vi "Reports_GetAllRequestsData.vi"(8 "error in (no error)":errorcluster, 11 "Refnum in":T1) -> (0 "error out":errorcluster, 2 "Array":string[][](array[string]), 3 "Refnum Out":T1)   [LabVIEW 2013, in "FIRST Reports.lvlib"]
uses:
  FIRST Reports.lvlib
  <vilib>/addons/database/Connection.llb/Conn ObjectReference.ctl
  Backend/source/VI Source/FRCts20_Backend_Engine.lvlib
  <vilib>/addons/database/NI_Database_API.lvlib
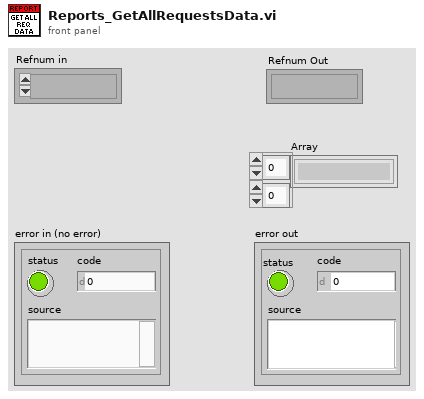
[diagram p1: front panel]
types:
  T1 = typedef "NI_Database_API.lvlib/Conn ObjectReference.ctl" = refnum<k1>
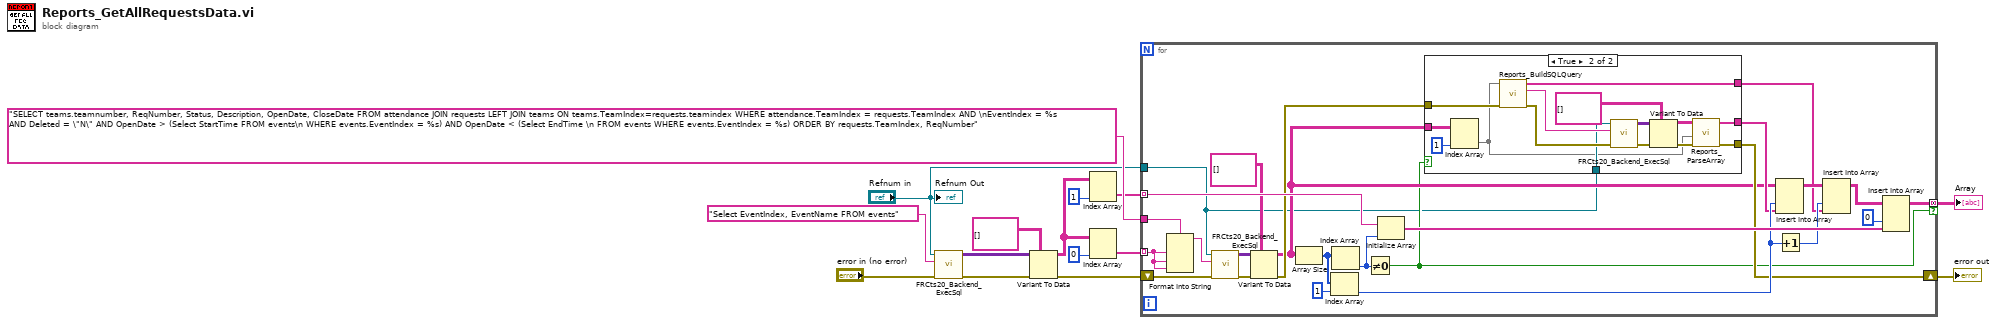
[diagram p0: block diagram]
diagram:
  n1 = call "FRCts20_Backend_ExecSql.vi"("error in (no error)"="error in (no error)", "format string"="Select EventIndex, EventName FROM events", "Refnum in"="Refnum in") -> ("error out"=w11:errorcluster, "recordset data"=w15:variant[][])  [unwired: 6 in, 1 out]
  n2 = Variant To Data(error in=w11, type=string[][] [], Variant=w15) -> (data=w9:string[][], error out=w4:errorcluster)
  n3 = Index Array(array=w9, index (col)=1 ("disabled index (col)")) -> (element=w7:string[])  [unwired: 1 in]
  n4 = Index Array(array=w9, index (col)=0 ("disabled index (col)")) -> (element=w12:string[])  [unwired: 1 in]
  n5 = for {
    tunnel: w12 -> [w39] mode=indexing
    tunnel: "Refnum in" -> [w16]
    tunnel: "SELECT teams.teamnumber, ReqNumber, Status, Description, OpenDate, CloseDate FROM attendance JOIN requests LEFT JOIN teams ON teams.TeamIndex=requests.teamindex WHERE attendance.TeamIndex = requests.TeamIndex AND \nEventIndex = %s AND Deleted = \"N\" AND OpenDate > (Select StartTime FROM events\n WHERE events.EventIndex = %s) AND OpenDate < (Select EndTime \n FROM events WHERE events.EventIndex = %s) ORDER BY requests.TeamIndex, ReqNumber" ("format string") -> [w40]
    tunnel: [w31] -> w5 mode=concatenating if=w18
    tunnel: w7 -> [w35] mode=indexing
    shift-right: [w20] -> w3
    shift-left: w4 -> [w17]
    n6 = Format Into String(format string=w40, w39, w39, w39) -> (resulting string=w38:string)  [unwired: 2 in, 1 out]
    n7 = call "FRCts20_Backend_ExecSql.vi"("error in (no error)"=w17, "format string"=w38, "Refnum in"=w16) -> ("error out"=w37:errorcluster, "recordset data"=w36:variant[][])  [unwired: 6 in, 1 out]
    n8 = Variant To Data(error in=w37, type=string[][] [], Variant=w36) -> (data=w19:string[][], error out=w22:errorcluster)
    n9 = Array Size(array=w19) -> (size(s)=w29:i32[])
    n10 = Index Array(array=w29, index=1) -> (element=w26:i32)
    n11 = Index Array(array=w29) -> (element=w30:i32)  [unwired: 1 in]
    n12 = Not Equal To 0?(x=w30) -> (x != 0?=w18:bool)
    n13 = Initialize Array(w35, w30) -> (w33:string[])
    n14 = case shown="True" w18 {
      tunnel: [_ w55] -> w24
      tunnel: w22 -> [w41 w54]
      tunnel: [_ w45] -> w21
      tunnel: [w41 w43] -> w20
      tunnel: w16 -> [_ w49]
      tunnel: w19 -> [_ w48]
      frame False {
      }
      frame True {
        n15 = Index Array(array=w48, index (col)=1 ("disabled index (col)")) -> (element=w42:string[])  [unwired: 1 in]
        n16 = call "Reports_BuildSQLQuery.vi"("error in (no error)"=w54, "Array of Event Indexes"=w42) -> ("error out"=w51:errorcluster, "SQL Query"=w50:string, "Array of Request URLs"=w55:string[])  [unwired: 7 in]
        n17 = call "FRCts20_Backend_ExecSql.vi"("error in (no error)"=w51, "format string"=w50, "Refnum in"=w49) -> ("error out"=w52:errorcluster, "recordset data"=w47:variant[][])  [unwired: 6 in, 1 out]
        n18 = Variant To Data(error in=w52, type=string[][] [], Variant=w47) -> (data=w46:string[][], error out=w44:errorcluster)
        n19 = call "Reports_ParseArray.vi"("error in (no error)"=w44, "Array Req#"=w42, "Array Req & Notes"=w46) -> ("error out"=w43:errorcluster, "Spaced Array"=w45:string[])  [unwired: 7 in]
      }
    }
    n20 = Insert Into Array(array=w19, index (col)=w26, new element=w21) -> (w27:string[][])  [unwired: 1 in]
    n21 = Increment(x=w26) -> (x+1=w25:i32)
    n22 = Insert Into Array(array=w27, index (col)=w25, new element=w24) -> (w23:string[][])  [unwired: 1 in]
    n23 = Insert Into Array(array=w23, index (col)=0 ("disabled index (col)"), new element=w33) -> (w31:string[][])  [unwired: 1 in]
  }
  "error out" <- w3
  "Array" <- w5
  "Refnum Out" <- "Refnum in"
